vi "G#SubSubClass2_SetModifiedAttributes.vi"(0 "reference in":refnum<class "G#SubSubClass2.lvclass">, 2 "attributes":T1, 3 "Only unlock data? (F)":bool, 4 "Unlock data if error? (T)":bool=TRUE, 5 "error in (no error)":errorcluster, 7 "Update data even if error? (F)":bool) -> (14 "reference out":refnum<class "G#SubSubClass2.lvclass">, 19 "error out":errorcluster)   [LabVIEW 2017, in "G#SubSubClass2.lvclass"]
doc: "This VI overwrites the class attributes associated with this class or subclass object reference and unlocks it for write access. If error in is set, the object is unlocked but its data will not be modified. If reference is wired, the class attributes of the class (or sub class) will be affected else the class attributes will default to the class.\n\nIn order to use this VI, you must first successfully lock the object's data using this class GetClassAttributesToModify VI."
uses:
  G#SubSubClass2.lvclass
  C:/Projects/GsharpGIT2017/Verification/TestCases/TestClasses/G#SubClass2_class/G#SubClass2.lvclass
  protected/ObjectAttributes.ctl
  G#SubClass2_class/protected/ObjectAttributes.ctl
  G#BaseClass2_class/protected/ObjectAttributes.ctl
  ObjectAttributesRef.ctl
  G#SubSubClass2.lvclass/G#SubSubClass2.ctl
  G#SubClass2_class/G#SubClass2.lvclass
  G#BaseClass2_class/G#BaseClass2.lvclass
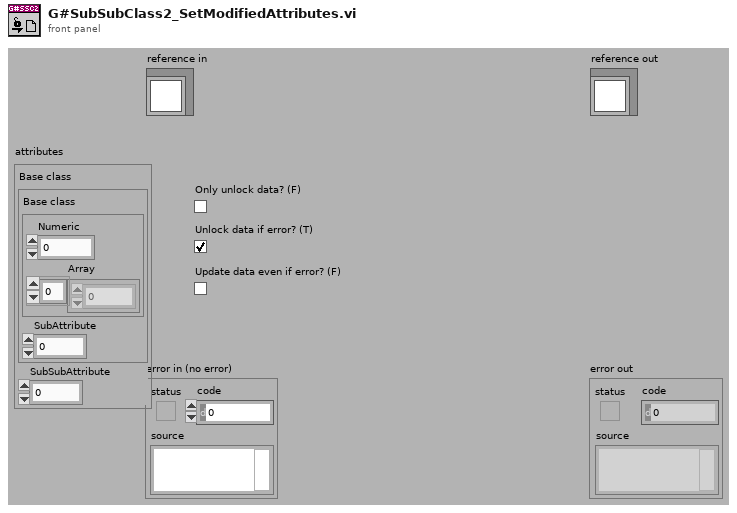
[diagram p1: front panel]
types:
  T1 = typedef "G#SubSubClass2.lvclass/ObjectAttributes.ctl" = cluster{"Base class":T2, "SubSubAttribute":dbl}
  T2 = typedef "G#SubClass2.lvclass/ObjectAttributes.ctl" = cluster{"Base class":T3, "SubAttribute":dbl}
  T3 = typedef "G#BaseClass2.lvclass/ObjectAttributes.ctl" = cluster{"Numeric":dbl, "Array":dbl[]}
  T4 = typedef "G#SubSubClass2.lvclass/ObjectAttributesRef.ctl" = refnum<data-value>
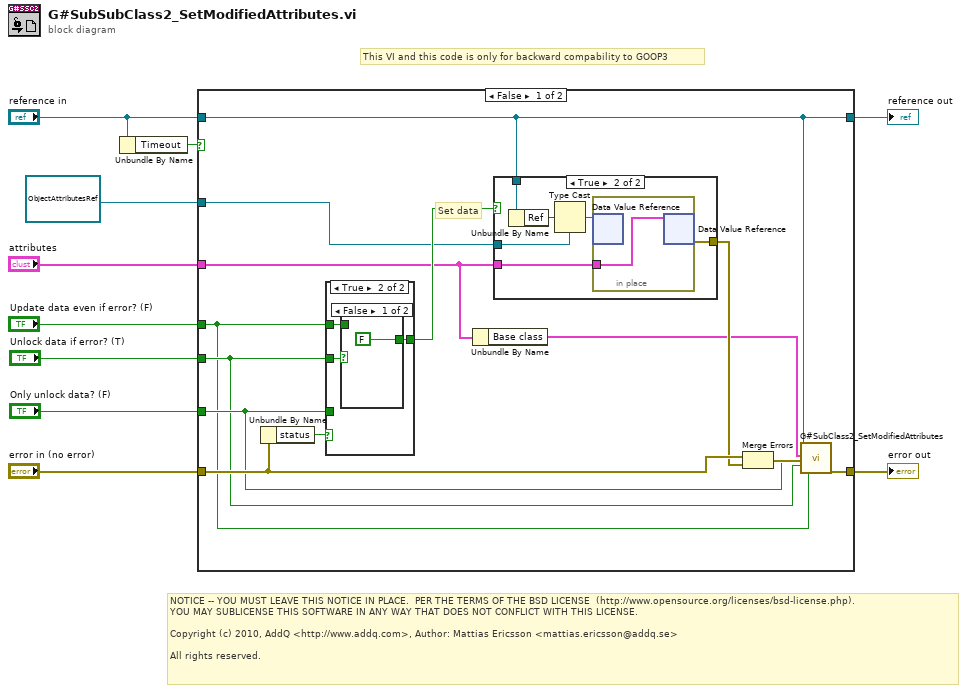
[diagram p0: block diagram]
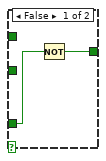
[diagram p3: hidden frame]
diagram:
  # "NOTICE -- YOU MUST LEAVE THIS NOTICE IN PLACE.  PER THE TERMS OF THE BSD LICENSE  (http://www.opensource.org/licenses/bsd-license.php).\nYOU MAY SUBLICENSE THIS SOFTWARE IN ANY WAY THAT DOES NOT CONFLICT WITH THIS LICENSE.\n\nCopyright (c) 2010, AddQ <http://www.addq.com>, Author: Mattias Ericsson <mattias.ericsson@addq.se>\n\nAll rights reserved."
  # "This VI and this code is only for backward compability to GOOP3"
  n1 = Unbundle By Name("reference in") -> ("Timeout"=w3:bool)
  n2 = case shown="False" w3 {
    tunnel: "error in (no error)" -> [w21 w38]
    tunnel: "attributes" -> [w18 _]
    tunnel: [w16 w38] -> w8
    tunnel: "Only unlock data? (F)" -> [w14 _]
    tunnel: "Unlock data if error? (T)" -> [w13 _]
    tunnel: "Update data even if error? (F)" -> [w12 _]
    tunnel: "reference in" -> [w15 w39]
    tunnel: [w15 w39] -> w2
    tunnel: T4 refnum ("attributes ref") -> [w11 _]
    frame False {
      # "Set data"
      n3 = Unbundle By Name(w21) -> ("status"=w23:bool)
      n4 = case shown="True" w23 {
        tunnel: [w31 w34] -> w22
        tunnel: w14 -> [w32 _]
        tunnel: w13 -> [_ w35]
        tunnel: w12 -> [_ w33]
        frame False {
          n5 = Not(x=w32) -> (.not. x?=w31:bool)
        }
        frame True {
          n6 = case shown="False" w35 {
            tunnel: [FALSE w37] -> w34
            tunnel: w33 -> [_ w37]
            frame False {
            }
            frame True {
            }
          }
        }
      }
      n7 = Unbundle By Name(w18) -> ("Base class"=w17:T2)
      n8 = case shown="True" w22 {
        tunnel: w18 -> [_ w29]
        tunnel: [_ w28] -> w20
        tunnel: w15 -> [_ w27]
        tunnel: w11 -> [_ w25]
        frame False {
        }
        frame True {
          n9 = Unbundle By Name(w27) -> ("Ref"=w26:u32)
          n10 = Type Cast(type=w25, x=w26) -> (*(type *) &x=w24:T4)
          n11 = in-place {
            in-place-border: w29 -> [w30]
            n12 = in-place-dvr #1(w24) -> ()  [unwired: 2 out]
            n13 = in-place-dvr #1(w30) -> (w28:errorcluster)  [unwired: 1 out]
          }
        }
      }
      n14 = Merge Errors(w21, w20) -> (w19:errorcluster)
      n15 = call "G#SubClass2_SetModifiedAttributes.vi"("reference in"=w15, "attributes"=w17, "Only unlock data? (F)"=w14, "Unlock data if error? (T)"=w13, "error in (no error)"=w19, "Update data even if error? (F)"=w12) -> ("error out"=w16:errorcluster)  [unwired: 12 in, 1 out]
    }
    frame True {
    }
  }
  "error out" <- w8
  "reference out" <- w2
